vi "Get Compiled Group Name and Type.vi"(10 "Channel Type":string, 11 "Group Name":string) -> (2 "Group Type":T1=enum."Input/Read", 3 "Computed Group Name":string)   [LabVIEW 2026, in "SystemMonitor Deployment Hooks.lvlib"]
uses:
  SystemMonitor Deployment Hooks.lvlib
  <vilib>/Utility/error.llb/Trim Whitespace (string).vi
  Types/Channel Mode.ctl
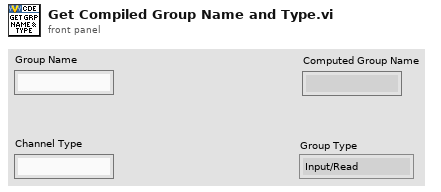
[diagram p1: front panel]
types:
  T1 = typedef "SystemMonitor Deployment Hooks.lvlib/Channel Mode.ctl" = enum16{"Output/Write", "Input/Read", "Input/ReadWrite"}
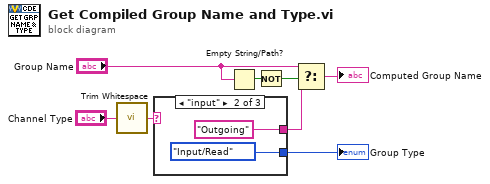
[diagram p0: block diagram]
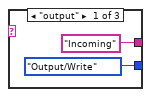
[diagram p2: hidden frame]
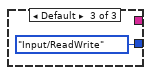
[diagram p3: hidden frame]
diagram:
  n1 = call-poly <vilib>:"Trim Whitespace.vi"("string"="Channel Type") -> ("trimmed string"=w1:string)  [unwired: 1 in]
  n2 = case shown="\"input\"" w1 {
    tunnel: [Channel_Mode."Output/Write" ("Channel Type") Channel_Mode."Input/Read" ("Channel Type") Channel_Mode."Input/ReadWrite" ("Channel Type")] -> w5
    tunnel: ["Incoming" "Outgoing" _] -> w8
    frame "output" {
    }
    frame "input" {
    }
    frame Default {
    }
  }
  "Group Type" <- w5
  n3 = Empty String/Path?(string/path="Group Name") -> (empty?=w7:bool)
  n4 = Not(x=w7) -> (.not. x?=w6:bool)
  n5 = Select(t="Group Name", s=w6, f=w8) -> (s? t:f=→"Computed Group Name":string)
